vi "RF Filter.vi"(8 "Error In":errorcluster, 9 "RF Signals In":waveform(dbl)[](array[waveform]), 10 "Type":enum16{"Bandpass", "AC", "No Filter"}(ring), 11 "IIR Filter Cluster in":T1) -> (0 "Error Out":errorcluster, 1 "Filtered Signals":waveform(dbl)[](array[waveform]))   [LabVIEW 2019]
uses:
  <vilib>/Analysis/3filter.llb/Zero Phase Filter (Cascade, DBL).vi
  <vilib>/Analysis/NI_AALBase.lvlib
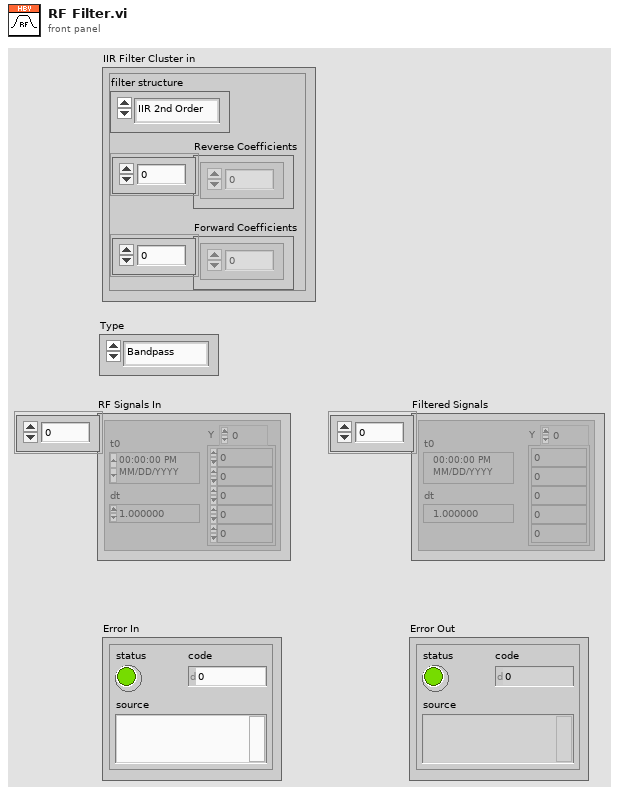
[diagram p1: front panel]
types:
  T1 = cluster{"filter structure":enum32{"IIR 2nd Order", "IIR 4th Order"}, "Reverse Coefficients":dbl[], "Forward Coefficients":dbl[]}
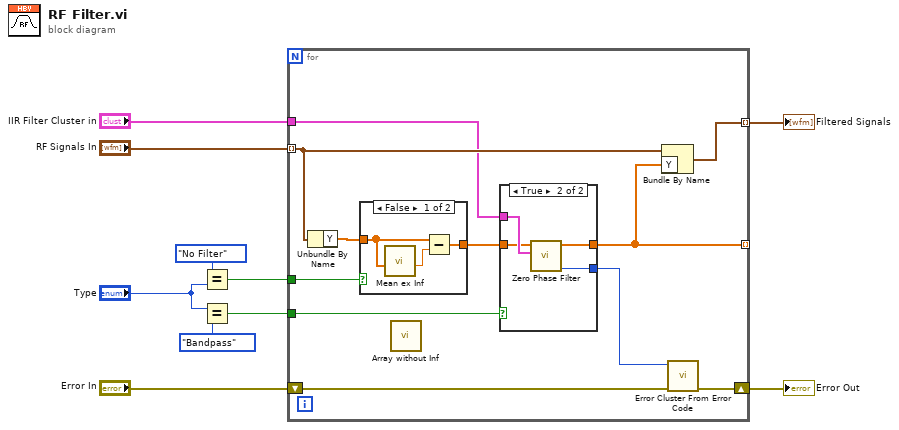
[diagram p0: block diagram]
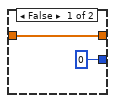
[diagram p2: hidden frame]
diagram:
  n1 = Equal?(x=enum16{"Bandpass", "AC", "No Filter"}."No Filter" ("y"), y="Type") -> (x = y?=w3:bool)
  n2 = Equal?(x="Type", y=enum16{"Bandpass", "AC", "No Filter"}."Bandpass") -> (x = y?=w1:bool)
  n3 = for {
    tunnel: w1 -> [w21]
    tunnel: w3 -> [w20]
    tunnel: "RF Signals In" -> [w17] mode=indexing
    tunnel: "IIR Filter Cluster in" -> [w11]
    tunnel: [w16] -> _ mode=indexing
    tunnel: [w15] -> w8 mode=indexing
    shift-right: [w14] -> w9
    shift-left: "Error In" -> [w13]
    n4 = Unbundle By Name(w17) -> ("Y"=w18:dbl[])
    n5 = case shown="False" w20 {
      tunnel: w18 -> [w29 w31]
      tunnel: [w30 w31] -> w19
      frame False {
        n6 = call "Mean ex Inf.vi"("Array"=w29) -> ("Mean ex Inf"=w28:dbl)  [unwired: 10 in]
        n7 = Subtract(x=w29, y=w28) -> (x-y=w30:dbl[])
      }
      frame True {
      }
    }
    n8 = call "Array without Inf.vi"() -> ()  [unwired: 11 in, 1 out]
    n9 = case shown="True" w21 {
      tunnel: [w23 w27] -> w16
      tunnel: [0 ("error") w26] -> w12
      tunnel: w11 -> [_ w25]
      tunnel: w19 -> [w23 w24]
      frame False {
      }
      frame True {
        n10 = call-poly <vilib>:"Zero Phase Filter.vi"("IIR Filter Cluster"=w25, "X"=w24) -> ("error"=w26:i32, "Filtered X"=w27:dbl[])  [unwired: 8 in]
      }
    }
    n11 = Bundle By Name(cluster=w17, "Y"=w16) -> (w15:waveform(dbl))
    n12 = call <vilib>:"Error Cluster From Error Code.vi"("error in (no error)"=w13, "error code (0)"=w12) -> ("error out"=w14:errorcluster)  [unwired: 7 in]
  }
  "Error Out" <- w9
  "Filtered Signals" <- w8
